vi "Reset.vi"(8 "Error In":errorcluster, 11 "OPI Ref":refnum<data-value>) -> (0 "Error Out":errorcluster, 3 "OPI Ref":refnum<data-value>)   [LabVIEW 2012, in "OPI.lvclass"]
doc: "Clear and remove all local argument lists. \n\nThis method does NOT remove any variables and functions defined in PES."
uses:
  OPI.lvclass
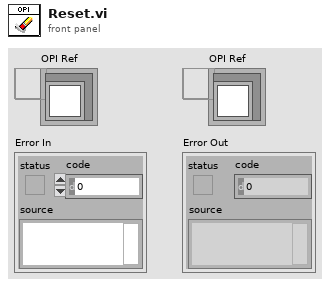
[diagram p1: front panel]
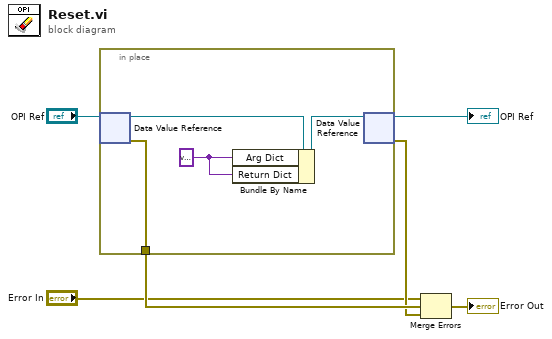
[diagram p0: block diagram]
diagram:
  n1 = in-place {
    in-place-border: [w7] -> w4
    w8 = variant ("Arg Dict")
    n2 = in-place-dvr #1("OPI Ref") -> (w10:refnum<class "OPI.lvclass">, w7:errorcluster)
    n3 = Bundle By Name(cluster=w10, "Arg Dict"=w8, "Return Dict"=w8) -> (w9:refnum<class "OPI.lvclass">)
    n4 = in-place-dvr #1(w9) -> (→"OPI Ref":refnum<data-value>, w3:errorcluster)
  }
  n5 = Merge Errors("Error In", w4, w3) -> (→"Error Out":errorcluster)
